vi "Agregar a listado.vi"(7 "Restar":refnum<vi>, 8 "error in (no error)":errorcluster, 9 "Restar?":bool, 10 "Listado":string[][](array[string]), 11 "Codigo":string) -> (0 "error out":errorcluster, 2 "Encontrado?":bool, 3 "Listado 2":string[][](array[string]))   [LabVIEW 2018]
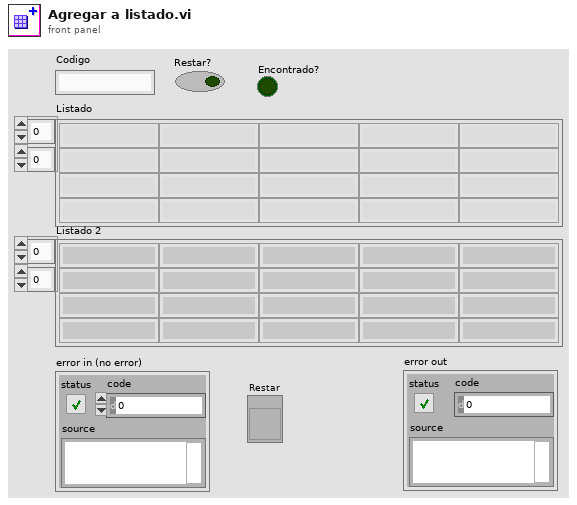
[diagram p1: front panel]
types:
  T1 = enum8{"Enabled", "Disabled", "Disabled and Grayed Out"}
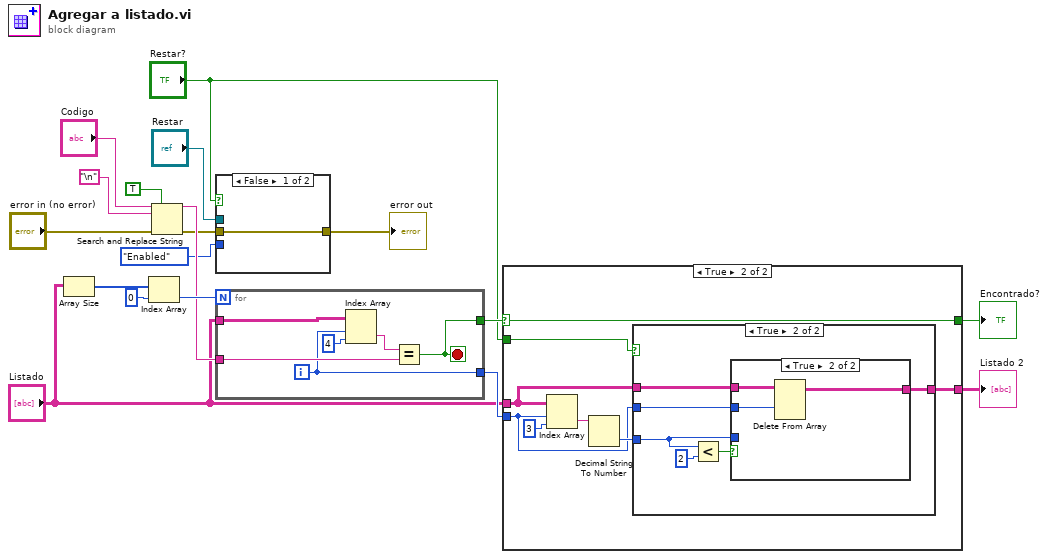
[diagram p0: block diagram]
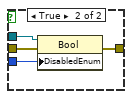
[diagram p2: hidden frame]
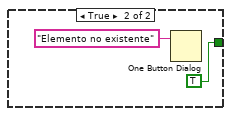
[diagram p4: hidden frame]
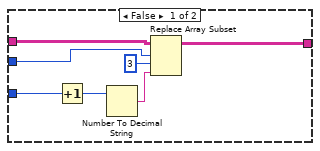
[diagram p5: hidden frame]
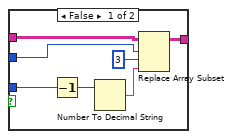
[diagram p6: hidden frame]
diagram:
  n1 = Array Size(array="Listado") -> (size(s)=w13:i32[])
  n2 = Index Array(array=w13, index=0) -> (element=w12:i32)
  n3 = Search and Replace String(replace all?=TRUE ("replace all? (F)"), input string="Codigo", search string="\n", error in="error in (no error)") -> (result string=w11:string, error out=w4:errorcluster)  [unwired: 4 in, 2 out]
  n4 = case shown="False" "Restar?" {
    tunnel: "Restar" -> [_ w23]
    tunnel: w4 -> [w19 w22]
    tunnel: [w19 w21] -> w3
    tunnel: T1."Enabled" ("Disabled") -> [_ w20]
    frame False {
    }
    frame True {
      n5 = property class="Bool"(reference=w23, error in=w22, "DisabledEnum"=w20) -> (error out=w21:errorcluster)  [unwired: 1 out]
    }
  }
  "error out" <- w3
  n6 = for {
    N: w12 -> [_]
    tunnel: w11 -> [w26]
    tunnel: "Listado" -> [w28]
    tunnel: [w25] -> w7
    tunnel: [w24] -> w10
    i -> [w24]
    stop <- w25 stop-if-true
    n7 = Index Array(array=w28, index (row)=w24, index (col)=4) -> (element=w27:string)
    n8 = Equal?(x=w27, y=w26) -> (x = y?=w25:bool)
  }
  n9 = case shown="True" w7 {
    selector: w7 -> [w31 w37]
    tunnel: w10 -> [_ w39]
    tunnel: "Listado" -> [w33 w40]
    tunnel: "Restar?" -> [w32 w42]
    tunnel: [w33 w38] -> w8
    tunnel: [w30 w37] -> w6
    frame False {
      n10 = case shown="False" w32 {
        tunnel: w31 -> [w34 _]
        tunnel: [w34 TRUE] -> w30
        frame False {
        }
        frame True {
          n11 = One Button Dialog(message="Elemento no existente") -> ()  [unwired: 1 in, 1 out]
        }
      }
    }
    frame True {
      n12 = Index Array(array=w40, index (row)=w39, index (col)=3 ("disabled index (col)")) -> (element=w43:string)
      n13 = Decimal String To Number(string=w43) -> (number=w41:i32)  [unwired: 2 in, 1 out]
      n14 = case shown="True" w42 {
        tunnel: w41 -> [w48 w53]
        tunnel: w40 -> [w49 w57]
        tunnel: w39 -> [w45 w54]
        tunnel: [w47 w52] -> w38
        frame False {
          n15 = Increment(x=w48) -> (x+1=w46:i32)
          n16 = Number To Decimal String(number=w46) -> (decimal integer string=w50:string)  [unwired: 1 in]
          n17 = Replace Array Subset(array=w49, new element=w50, index (row)=w45, index (col)=3 ("disabled index (col)")) -> (w47:string[][])
        }
        frame True {
          n18 = Less?(x=w53, y=2) -> (x < y?=w56:bool)
          n19 = case shown="True" w56 {
            tunnel: w57 -> [w64 w67]
            tunnel: [w63 w66] -> w52
            tunnel: w54 -> [w62 w65]
            tunnel: w53 -> [w61 _]
            frame False {
              n20 = Decrement(x=w61) -> (x-1=w59:i32)
              n21 = Number To Decimal String(number=w59) -> (decimal integer string=w58:string)  [unwired: 1 in]
              n22 = Replace Array Subset(array=w64, new element=w58, index (row)=w62, index (col)=3 ("disabled index (col)")) -> (w63:string[][])
            }
            frame True {
              n23 = Delete From Array(array=w67, index (row)=w65) -> (array with subset deleted=w66:string[][])  [unwired: 2 in, 1 out]
            }
          }
        }
      }
    }
  }
  "Encontrado?" <- w6
  "Listado 2" <- w8
